vi "Read Address.vi"(11 "Network Stream in":refnum<class "Network Stream.lvclass">) -> (2 "Address":string)   [LabVIEW 2023, in "Network Stream.lvclass"]
uses:
  Network Stream.lvclass
  Network Stream.lvclass/Network Stream.ctl
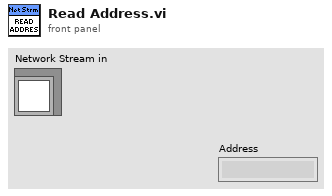
[diagram p1: front panel]
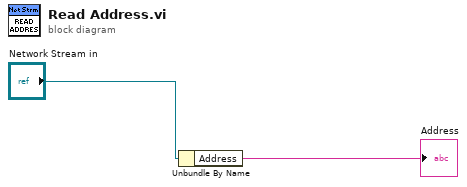
[diagram p0: block diagram]
diagram:
  n1 = Unbundle By Name("Network Stream in") -> ("Address"=→"Address":string)
